vi "AO redefine.vi"(6 "conninfo":T3={"host"="localhost", "port"="5432", "client_encoding"="WIN1251", "dbname"="data", "user"="postgres", "password"=""}, 7 "KFM":string[](array[string]), 8 "error in (no error)":errorcluster, 9 "AOParamTable":string="fao_3", 10 "AOParameters":string[](array[string]), 11 "AO in":T1) -> (0 "error":errorcluster, 3 "AO out":T1)   [LabVIEW 2019, in "Inputs.lvlib"]
uses:
  Inputs.lvlib
  Ctl/AO.ctl
  Ctl/Parameter State.ctl
  Database/ctl/Coninfo.ctl
  Ctl/AOParamColumns.ctl
  Database/PostgreSQL2LabVIEW/libpqUtility/src/PQconnect.vi
  Database/PostgreSQL2LabVIEW/libpqUtility/src/PQclose.vi
  Database/select_initial_all.vi
  Database/PostgreSQL2LabVIEW/libpqlv/src/PQfinish.vi
  Database/PostgreSQL2LabVIEW/libpqlv/src/PQconnectdb.vi
  Database/PostgreSQL2LabVIEW/libpqlv/src/PQerrorMessage.vi
  Database/PostgreSQL2LabVIEW/libpqlv/src/PQstatus.vi
  <vilib>/dlg_ctls.llb/Space Constant.vi
  Database/PostgreSQL2LabVIEW/libpqUtility/src/PQgetTable.vi
  Database/Progress.vi
  Database/PostgreSQL.lvlib
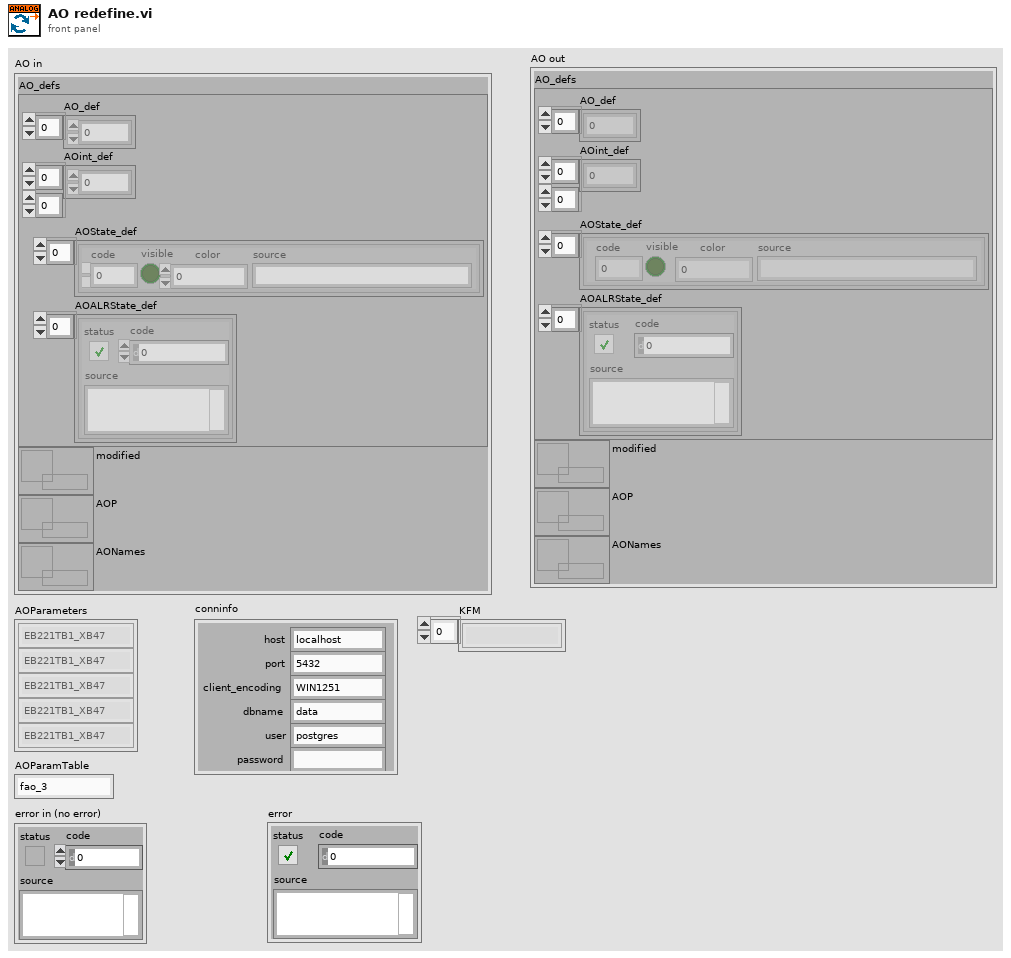
[diagram p1: front panel]
types:
  T1 = typedef "Inputs.lvlib/AO.ctl" = cluster{"AO_defs":cluster{"AO_def":dbl[], "AOint_def":u16[][], "AOState_def":T2[], "AOALRState_def":errorcluster[]}, "modified":refnum<data-value>, "AOP":refnum<data-value>, "AONames":refnum<data-value>}
  T2 = typedef "Inputs.lvlib/Parameter State.ctl" = cluster{"code":i32, "visible":bool, "color":u32, "source":string}
  T3 = typedef "PostgreSQL.lvlib/Coninfo.ctl" = cluster{"host":string, "port":string, "client_encoding":string, "dbname":string, "user":string, "password":string}
  T4 = typedef "Inputs.lvlib/AOParamColumns.ctl" = enum16{"instrument_gain", "instrument_offset", "instrument_range_min", "instrument_range_max", "output_pv_min", "output_pv_max", "output_register_min", "output_register_max", "module_fcode_full", "control_channel_num", "fcode", "fcodef", "fcode_full", "fname", "instrument_units"}
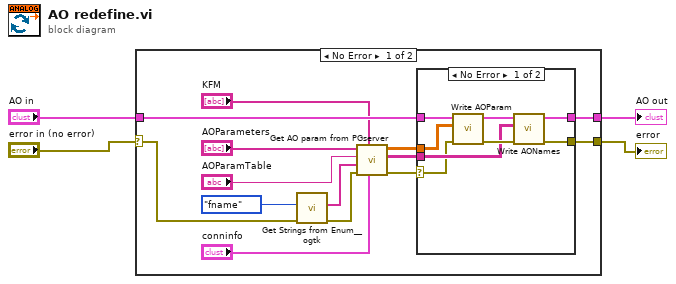
[diagram p0: block diagram]
diagram:
  n1 = case shown="No Error" "error in (no error)" {
    selector: "error in (no error)" -> [w6 w30]
    tunnel: [w13 w30] -> w4
    tunnel: "AO in" -> [w11 w29]
    tunnel: [w10 w29] -> w3
    frame No Error {
      n2 = call <userlib>:"Get Strings from Enum__ogtk.vi"("error in (no error)"=w6, "Enum"=AOParamColumns."fname" ("AOParamColumns")) -> ("error out"=w5:errorcluster, "Enum Strings"=w7:string[])  [unwired: 6 in, 2 out]
      n3 = call "Get AO param from PGserver.vi"("conninfo"="conninfo", "KFM"="KFM", "error in (no error)"=w5, "AOParamColumns"=w7, "AOParamTable"="AOParamTable", "AO_fcode_full"="AOParameters") -> ("error out"=w15:errorcluster, "Names table"=w16:string[][], "Parameters table"=w17:dbl[][])  [unwired: 3 in]
      n4 = case shown="No Error" w15 {
        selector: w15 -> [w19 w27]
        tunnel: w17 -> [w20 _]
        tunnel: w16 -> [w21 _]
        tunnel: [w23 w27] -> w13
        tunnel: w11 -> [w26 w28]
        tunnel: [w22 w28] -> w10
        frame No Error {
          n5 = call "Write AOParam.vi"("error in (no error)"=w19, "AOParam"=w20, "AO in"=w26) -> ("error out"=w24:errorcluster, "AO out"=w25:T1)  [unwired: 7 in]
          n6 = call "Write AONames.vi"("error in (no error)"=w24, "AONames"=w21, "AO in"=w25) -> ("error out"=w23:errorcluster, "AO out"=w22:T1)  [unwired: 7 in]
        }
        frame Error {
        }
      }
    }
    frame Error {
    }
  }
  "AO out" <- w3
  "error" <- w4
